vi "Properties To Create.vi"(8 "error in (no error)":errorcluster, 11 "CD Template in":refnum<class "NIVS_Inline HW Interface (Inline-Async).lvclass">) -> (0 "error out":errorcluster, 2 "Properties":T1[](array[typedef]))   [LabVIEW 2017, in "NIVS_Inline HW Interface (Inline-Async).lvclass"]
uses:
  NIVS_Inline HW Interface (Inline-Async).lvclass
  NIVS_Consolidated_CDW_MetaDataObj/Property Information.ctl
  NIVS_Consolidated_CDW_MetaDataObj/NIVS_Consolidated_CDW_MetaDataObj.lvclass
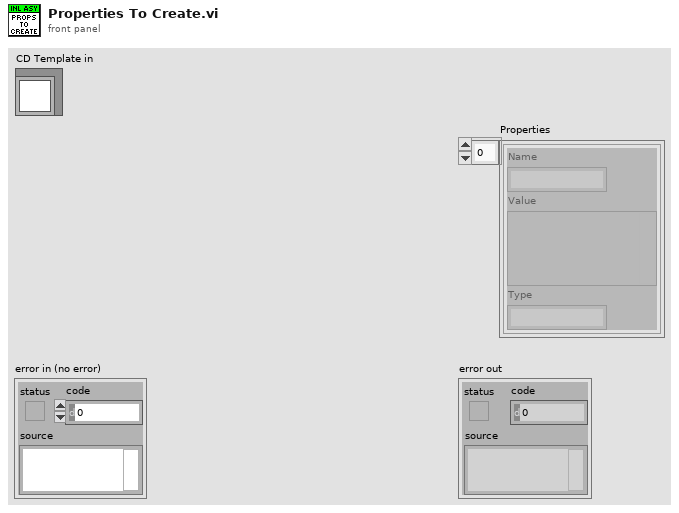
[diagram p1: front panel]
types:
  T1 = typedef "NIVS_Consolidated_CDW_MetaDataObj.lvclass/Property Information.ctl" = cluster{"Name":string, "Value":variant, "Type":string}
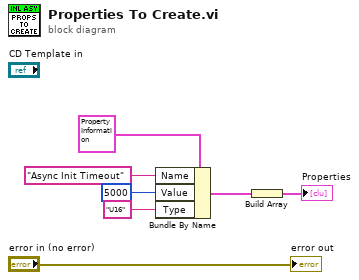
[diagram p0: block diagram]
diagram:
  n1 = Bundle By Name(cluster=T1 {"Name"="", "Value"=variant, "Type"=""} ("Property Info"), "Name"="Async Init Timeout", "Value"=u16 5000, "Type"="U16") -> (w2:T1)
  n2 = Build Array(w2) -> (→"Properties":T1[])
  "error out" <- "error in (no error)"
